vi "Setup Loop Iterator.vi"(6 "Loop":cluster{i32, i32}(slide)={0, 2}, 8 "error in (no error)":errorcluster, 9 "Total Loops":i32, 10 "Loop Iterator":u32, 11 "Previous Line":i32) -> (0 "error out":errorcluster, 1 "First Loop Out":bool, 2 "Loop Iterator Out":u32, 3 "Line Iterator Out":i32, 4 "Start Of Loop Out":bool, 5 "Inside Loop Out":bool)   [LabVIEW 2018, in "Multi Segment Waveform.xctl"]
doc: "Works out if the current instruction being processed is inside a loop or not."
uses:
  Multi Segment Waveform.xctl
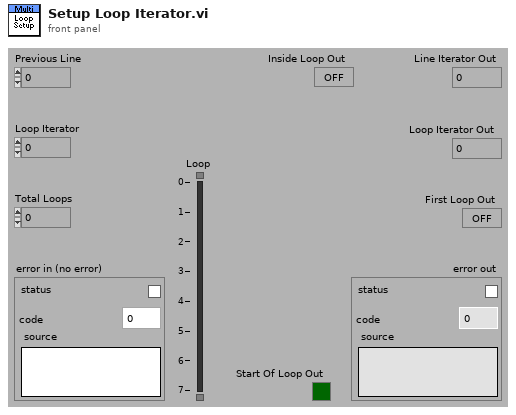
[diagram p1: front panel]
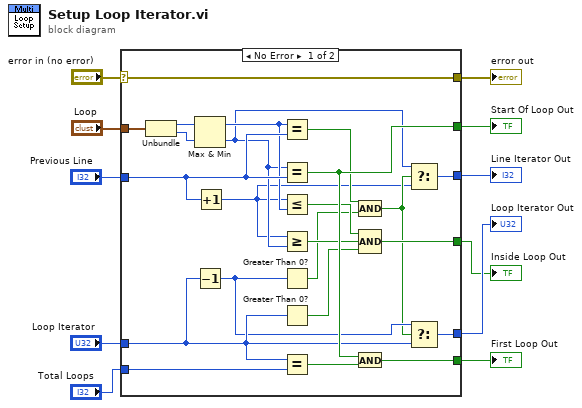
[diagram p0: block diagram]
diagram:
  n1 = case shown="No Error" "error in (no error)" {
    selector: "error in (no error)" -> [w25 w35]
    tunnel: [w34 _] -> w11
    tunnel: [w33 _] -> w10
    tunnel: "Loop" -> [w32 _]
    tunnel: [w31 _] -> w8
    tunnel: "Total Loops" -> [w30 _]
    tunnel: [w29 _] -> w6
    tunnel: [w28 _] -> w5
    tunnel: "Loop Iterator" -> [w27 _]
    tunnel: "Previous Line" -> [w26 _]
    tunnel: [w25 w35] -> w2
    frame No Error {
      n2 = Unbundle(w32) -> (w22:i32, w21:i32)
      n3 = Max & Min(x=w22, y=w21) -> (max(x,y)=w19:i32, min(x,y)=w16:i32)
      n4 = Decrement(x=w27) -> (x-1=w24:u32)
      n5 = Increment(x=w26) -> (x+1=w13:i32)
      n6 = Equal?(x=w19, y=w26) -> (x = y?=w23:bool)
      n7 = Equal?(x=w16, y=w26) -> (x = y?=w29:bool)
      n8 = Less Or Equal?(x=w13, y=w19) -> (x <= y?=w17:bool)
      n9 = Greater Or Equal?(x=w13, y=w16) -> (x >= y?=w18:bool)
      n10 = Greater Than 0?(x=w24) -> (x > 0?=w15:bool)
      n11 = Greater Than 0?(x=w27) -> (x > 0?=w14:bool)
      n12 = Equal?(x=w27, y=w30) -> (x = y?=w12:bool)
      n13 = And(x=w29, y=w12) -> (x .and. y?=w28:bool)
      n14 = Compound Arithmetic op=AND(w23, w15) -> (w20:bool)
      n15 = Compound Arithmetic op=AND(w17, w18, w14) -> (w31:bool)
      n16 = Select(t=w16, s=w20, f=w13) -> (s? t:f=w34:i32)
      n17 = Select(t=w24, s=w20, f=w27) -> (s? t:f=w33:u32)
    }
    frame Error {
    }
  }
  "Inside Loop Out" <- w8
  "Line Iterator Out" <- w11
  "Loop Iterator Out" <- w10
  "Start Of Loop Out" <- w6
  "First Loop Out" <- w5
  "error out" <- w2
